vi "一体站氨氮总磷流程平行样自动启动.vi"(11 "参数":T1) -> ()   [LabVIEW 2016, in "质控单元.lvlib"]
panel:
  out "枚举":enum16{"初始化", "采配水启动", "等待", "配水", "排水", "结束"}(ring)
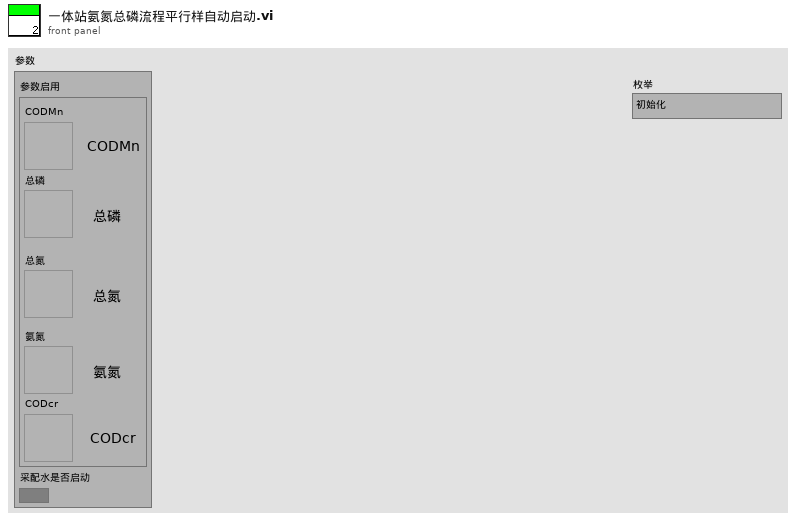
[diagram p1: front panel]
types:
  T1 = cluster{"参数启用":cluster{"CODMn":bool, "总磷":bool, "总氮":bool, "氨氮":bool, "CODcr":bool}, "采配水是否启动":bool}
  T2 = cluster{"命令":string, cluster{"starting address":u16, "holding register value":u16}}
  T3 = typedef "质控单元.lvlib/平行样测试流程.ctl" = enum16{"待机", "第一次水样测试启动", "第一次水样测试中", "第二次水样测试启动", "第二次水样测试中", "存储平行样测试数据", "结束"}
  T4 = cluster{"站号":u16, "量程切换":enum32{"H", "L", "AUTO"}, "控制命令":enum16{"启动测量", "标样核查", "零点核查", "跨度核查", "空白测试", "平行样测试", "加标回收", "空白校准", "标样校准", "初始化（清洗）", "停止测试", "仪器重启", "校时", "模式设置", "测量间隔设置"}, "模式设置":enum16{"待机", "连续模式", "周期模式", "定点模式", "受控模式", "手动模式"}, "测量间隔":u16}
  T5 = cluster{"时间标识":timestamp, "设备":string, "日志信息":string}
  T6 = enum16{"空闲", "水样测试", "标样核查", "零点核查", "跨度核查", "空白测试", "平行样测试", "加标回收", "空白校准", "标样校准", "初始化（清洗）"}
  T7 = cluster{"测量模式":enum16{"水样测量", "标样核查", "零点核查", "跨度核查", "空白测试", "加标回收", "平行样", "校零", "校标"}}
  T8 = cluster{"时间标识":timestamp, "设备":string, "日志信息":string, "流程参数":string}
  T9 = cluster{"R0":i16, "R1":i16, "R2":i16, "R3":i16, "R4":i16, "R5":i16, "R6":i16, "R7":i16, "R8":i16, "R9":i16, "R10":i16, "R11":i16, "R12":i16, "R13":i16, "R14":i16, "R15":i16, "R16":i16, "R17":i16, "R18":i16, "R19":i16, "R20":i16, "R21":i16, "R22":i16, "R23":i16, "R24":i16, "R25":i16, "R26":i16, "R27":i16, "R28":i16, "R29":i16, "R30":i16, "R31":i16, "R32":i16, "R33":i16, "R34":i16, "R35":i16, "R36":i16, "R37":i16, "R38":i16, "R39":i16, "R40":i16, "R41":i16, "R42":i16, "R43":i16, "R44":i16, "R45":i16, "R46":i16, "R47":i16, "R48":i16, "R49":i16, "R50":i16, "R51":i16, "R52":i16, "R53":i16, "R54":i16, "R55":i16, "R56":i16}
  T10 = cluster{"系统时间":timestamp, "工作状态":enum16{"空闲", "水样测试", "标样核查", "零点核查", "跨度核查", "空白测试", "平行样测试", "加标回收", "空白校准", "标样校准", "初始化（清洗）"}, "测量模式":enum16{"待机", "连续模式", "周期模式", "定点模式", "受控模式", "手动模式"}, "告警代码":enum16{"无告警", "缺试剂告警", "缺水样告警", "缺蒸馏水告警", "缺标液告警", "仪表漏液告警", "标定异常告警", "超量程告警", "加热异常", "低试剂预警", "超上限告警", "超下限告警", "仪表内部其他异常", "滴定异常告警", "电极异常告警", "量程切换告警", "参数设置告警", "PH电极电位异常", "电导率电极异常", "浊度光度异常", "溶解氧电极异常", "溶解氧光强异常", "温度异常告警", "PH异常告警", "溶解氧异常告警", "电导率异常告警", "浊度异常告警", "叶绿素异常告警", "藻密度异常告警", "蓝绿藻异常告警", "ORP异常告警", "氨氮异常告警", "清洁刷异常告警", "SD卡异常告警", "蓝牙异常告警", "Wifi异常告警", "流程异常告警"}, "故障代码":enum16{"无故障", "电机故障", "温度故障", "通讯故障", "滴定故障"}, "日志代码":u16, "软件版本":u16, "F0":sgl, "F1":sgl, "F2":sgl, "F3":sgl, "T":sgl, "H":sgl, "id":u16, "flowid":u16, "量程":u16, "总磷控温温度1":sgl, "营养盐控温温度2":sgl, "ADC":sgl}
  T11 = cluster{"因子编码":u32, "单位":u16, "标样参考值":sgl, "水样数据时间":timestamp, "水样实测值":sgl, "水样数据标识":string, "标样数据时间":timestamp, "标样实测值":sgl, "标样数据标识":string, "空白数据时间":timestamp, "空白实测值":sgl, "空白数据标识":string, "零点核查数据时间":timestamp, "零点核查实测值":sgl, "零点核查数据标识":string, "跨度核查数据时间":timestamp, "跨度核查实测值":sgl, "跨度核查数据标识":string, "加标回收数据时间":timestamp, "加标回收实测值":sgl, "加标回收数据标识":string, "平行样数据时间":timestamp, "平行样实测值":sgl, "平行样数据标识":string}
  T12 = cluster{"时间标识":timestamp, "参数":string, "数据类型":string, "第一次水样浓度值":sgl, "第二次水样测试时间":timestamp, "第二次水样浓度值":sgl}
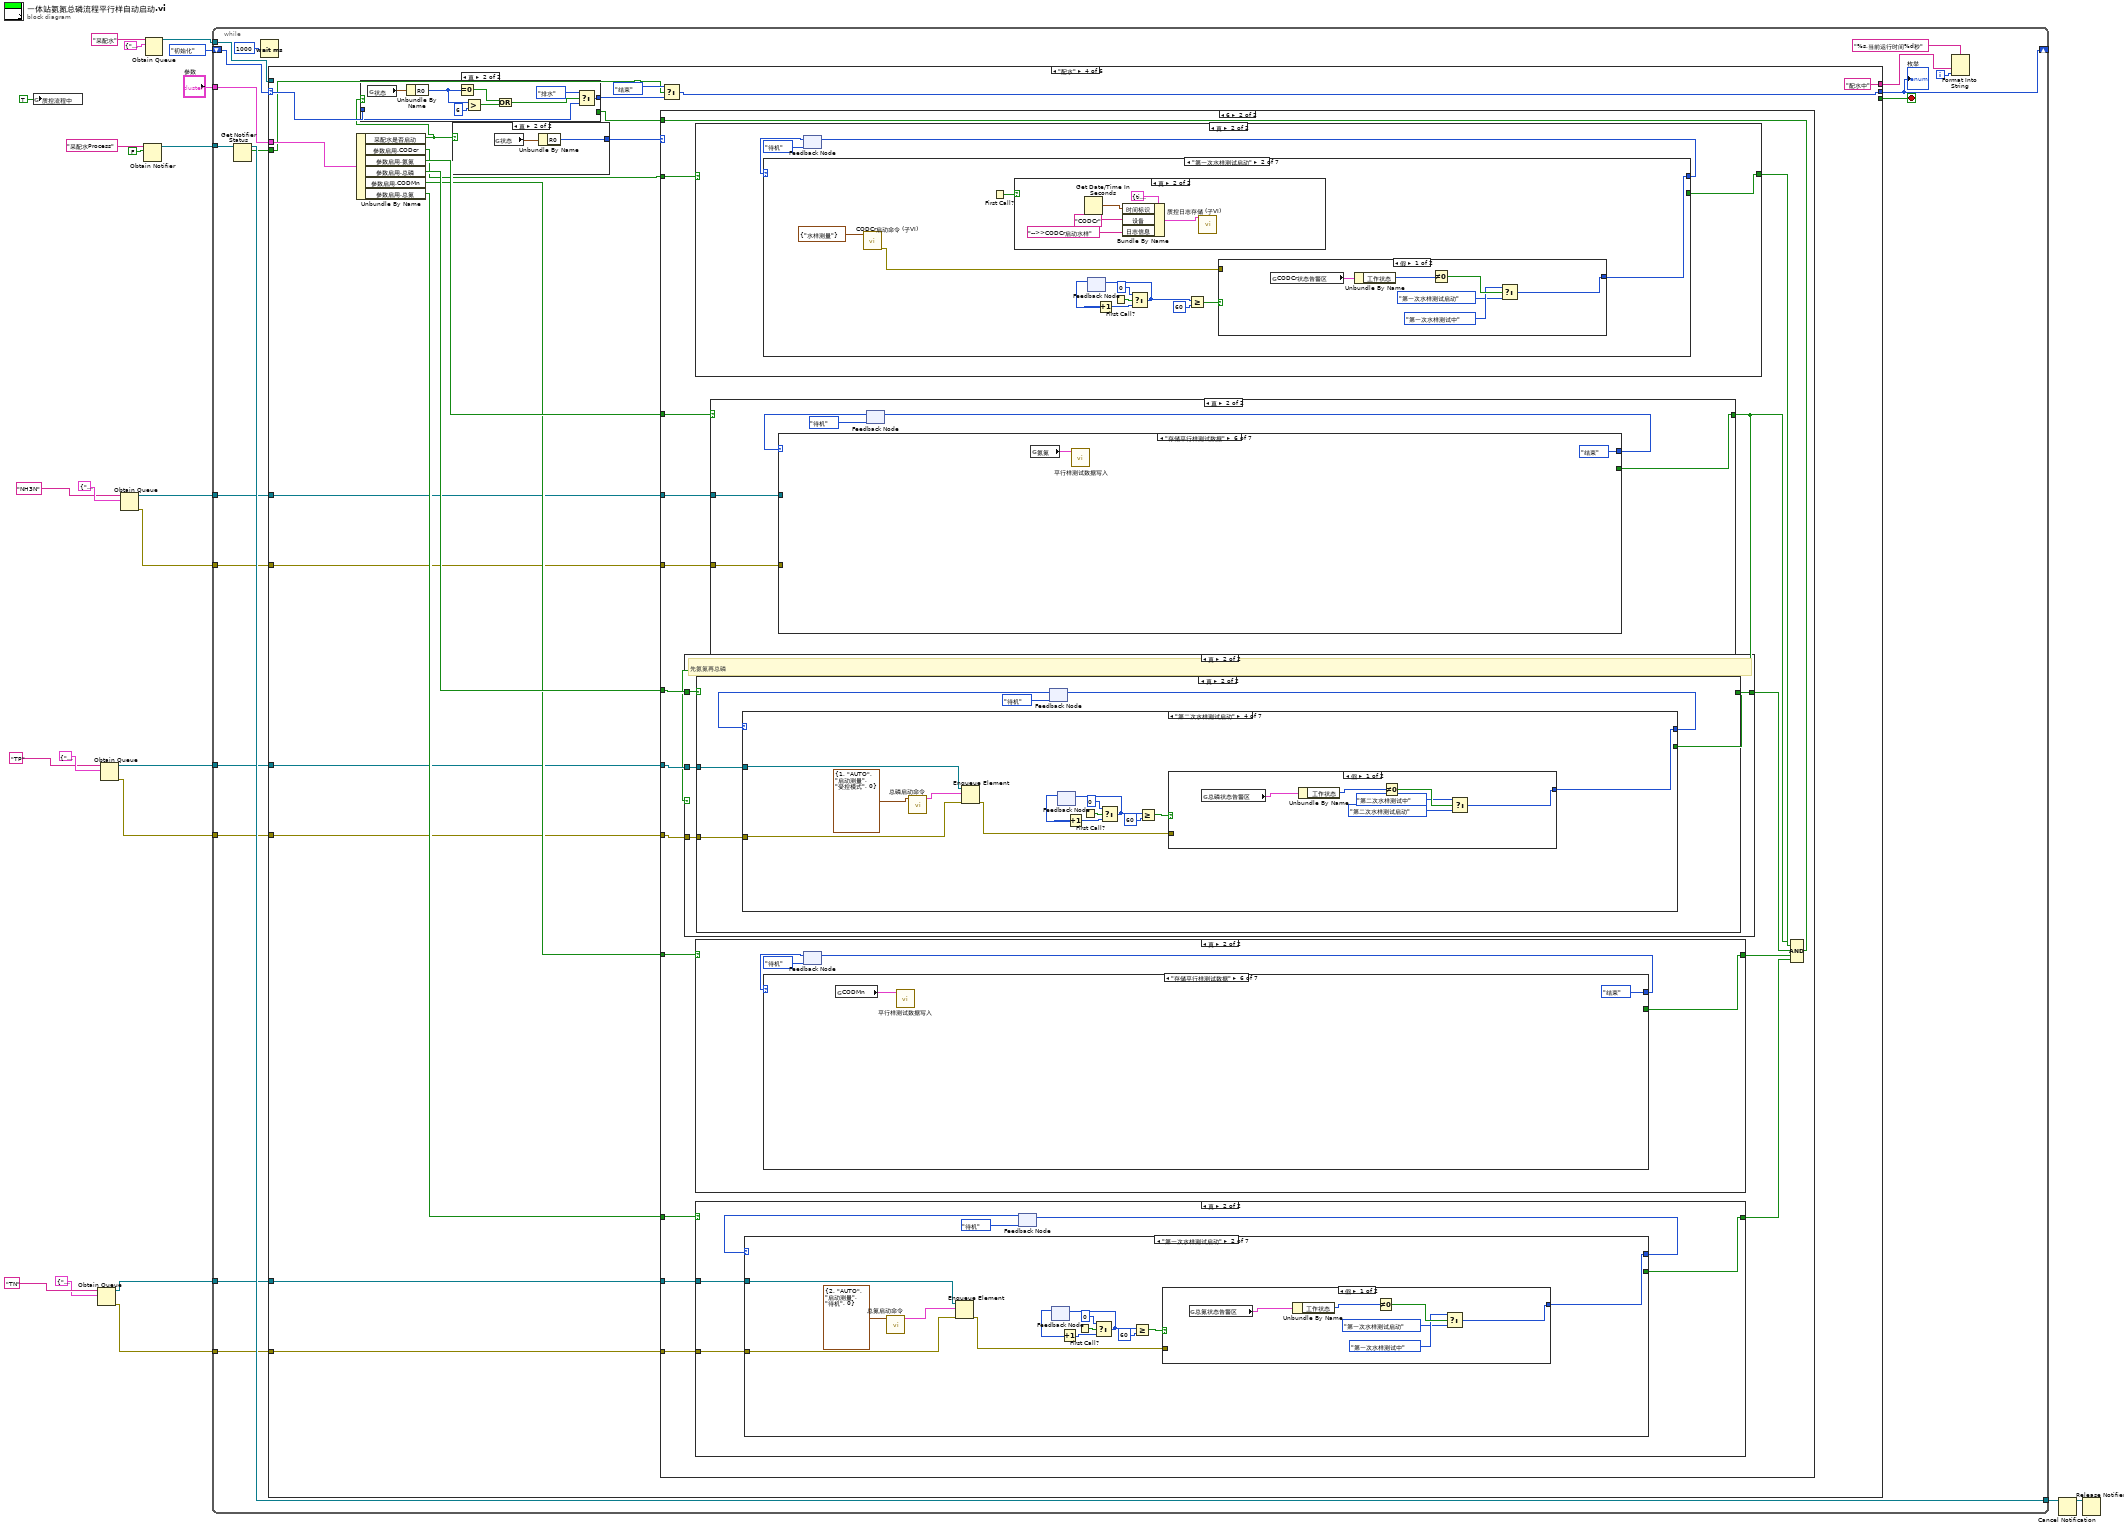
[diagram p0: block diagram]
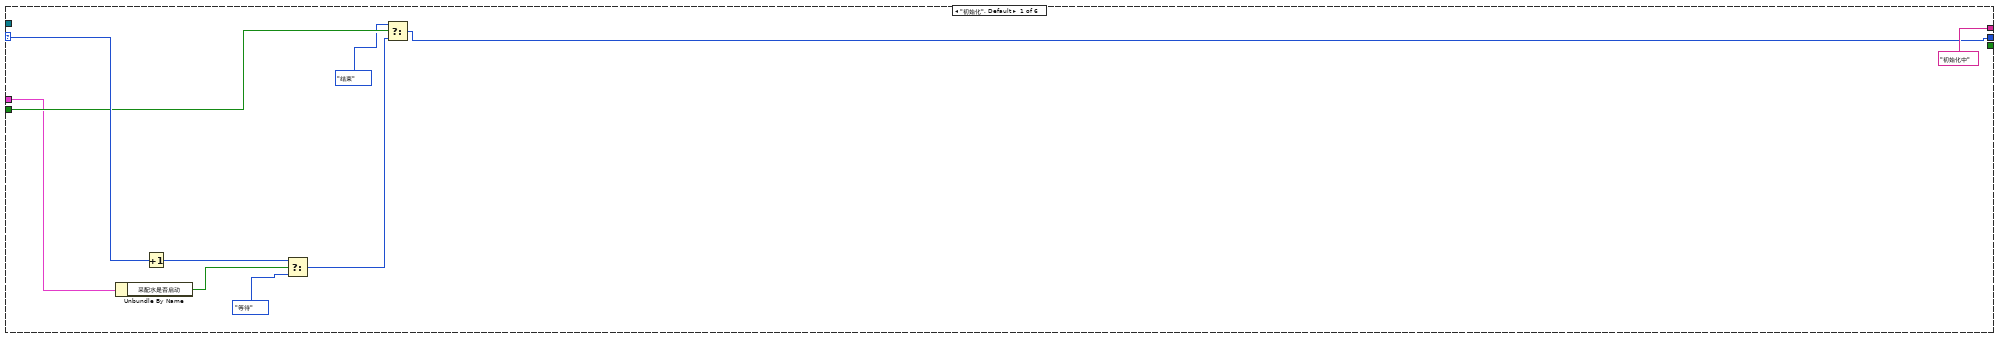
[diagram p2: hidden frame]
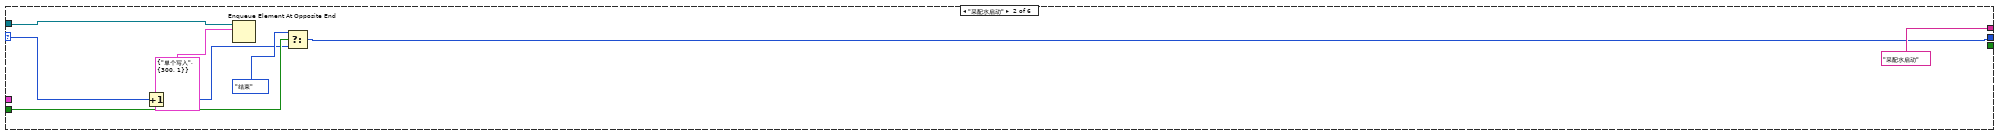
[diagram p3: hidden frame]
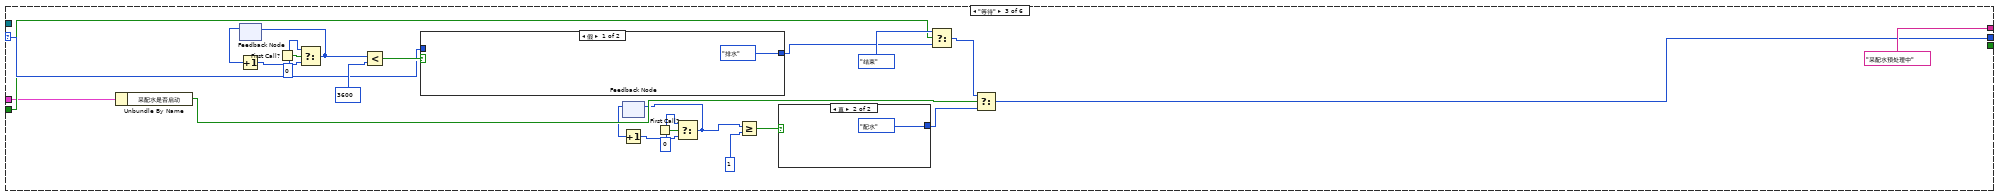
[diagram p4: hidden frame]
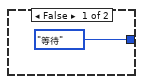
[diagram p5: hidden frame]
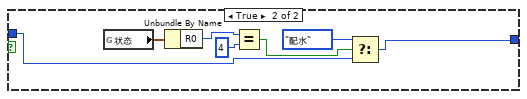
[diagram p6: hidden frame]
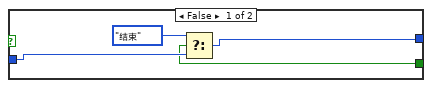
[diagram p7: hidden frame]
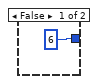
[diagram p8: hidden frame]
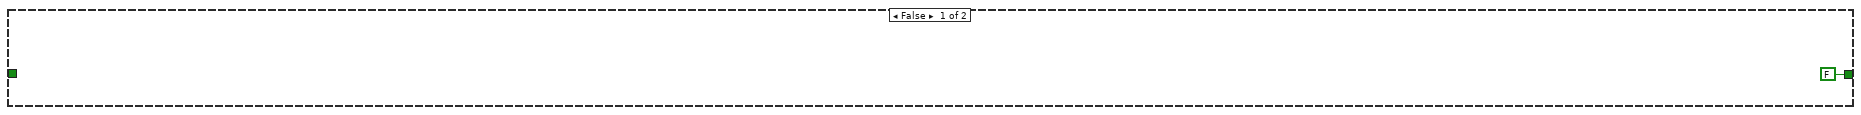
[diagram p10: hidden frame]
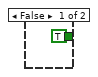
[diagram p11: hidden frame]
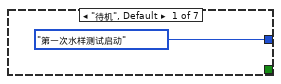
[diagram p12: hidden frame]
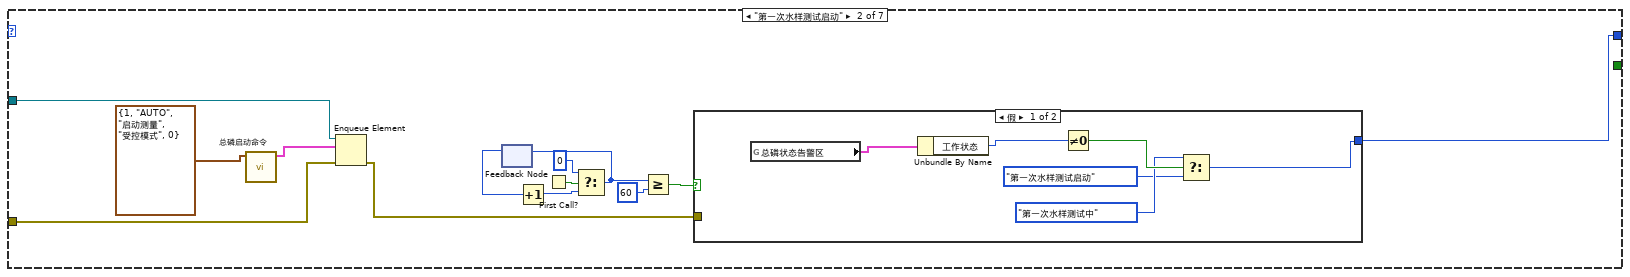
[diagram p13: hidden frame]
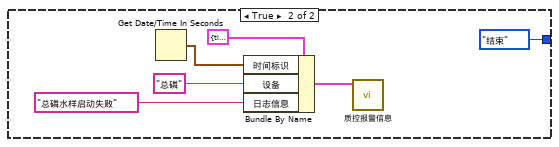
[diagram p14: hidden frame]
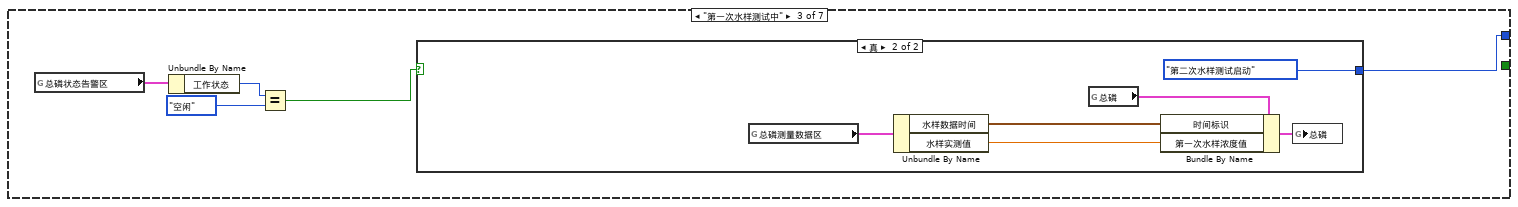
[diagram p15: hidden frame]
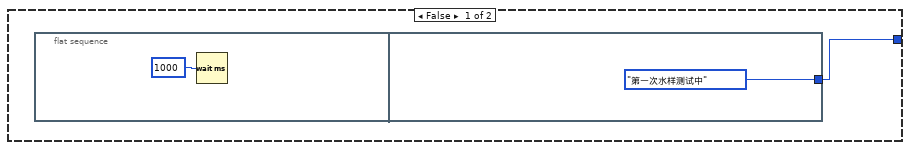
[diagram p16: hidden frame]
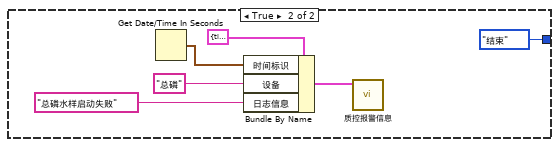
[diagram p17: hidden frame]
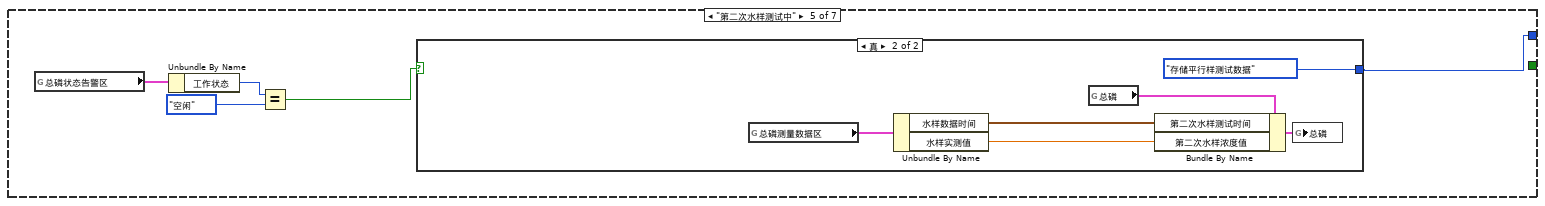
[diagram p18: hidden frame]
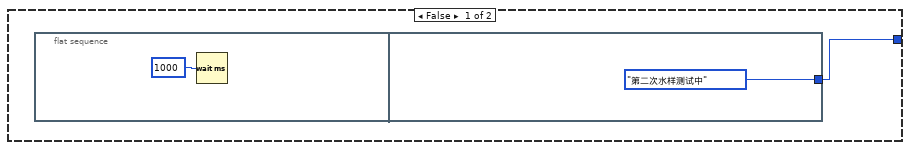
[diagram p19: hidden frame]
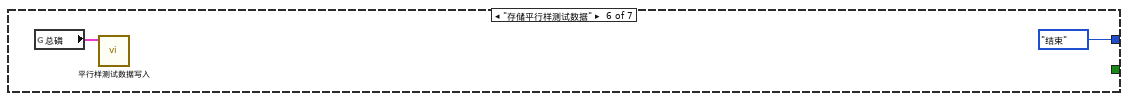
[diagram p20: hidden frame]
diagram:
  n1 = global write "质控测完标志全局 1.vi" "质控流程中"(TRUE ("质控流程中")) -> ()
  n2 = Obtain Queue(name (unnamed)="TN" ("名称（未命名）"), element data type=cluster{"命令":string, "data":variant} {"命令"="", "data"=variant}) -> (queue out=w3:refnum<queue>, error out=w2:errorcluster)  [unwired: 3 in, 1 out]
  n3 = Obtain Queue(name (unnamed)="TP" ("名称（未命名）"), element data type=cluster{"命令":string, "data":variant} {"命令"="", "data"=variant}) -> (queue out=w5:refnum<queue>, error out=w4:errorcluster)  [unwired: 3 in, 1 out]
  n4 = Obtain Queue(name (unnamed)="NH3N" ("名称（未命名）"), element data type=cluster{"命令":string, "data":variant} {"命令"="", "data"=variant}) -> (queue out=w7:refnum<queue>, error out=w6:errorcluster)  [unwired: 3 in, 1 out]
  n5 = Obtain Notifier(name (unnamed)="采配水Process" ("名称（未命名）"), notification data type=FALSE) -> (notifier out=w16:refnum<notifier>)  [unwired: 2 in, 2 out]
  n6 = Obtain Queue(name (unnamed)="采配水" ("名称（未命名）"), element data type=cluster{"命令":string, "数据":variant} {"命令"="", "数据"=variant}) -> (queue out=w21:refnum<queue>)  [unwired: 3 in, 2 out]
  n7 = while {
    tunnel: w21 -> [w41]
    shift-right: [w39] -> _
    shift-left: enum16{"初始化", "采配水启动", "等待", "配水", "排水", "结束"}."初始化" ("枚举") -> [w40]
    tunnel: "参数" -> [w37]
    tunnel: w16 -> [w36]
    tunnel: [w35] -> w15
    tunnel: w7 -> [w30]
    tunnel: w6 -> [w29]
    tunnel: w5 -> [w28]
    tunnel: w4 -> [w27]
    tunnel: w3 -> [w26]
    tunnel: w2 -> [w25]
    i -> [w32]
    stop <- w24 stop-if-true
    n8 = Get Notifier Status(notifier=w36) -> (notifier out=w35:refnum<notifier>, current notification=w31:bool)  [unwired: 1 in, 3 out]
    n9 = Wait (ms)(milliseconds to wait=u32 1000 ("等待时间（毫秒）")) -> ()  [unwired: 1 out]
    n10 = case shown="\"配水\"" w40 {
      selector: w40 -> [w51 w57 w81 w114 w596 w603]
      tunnel: w41 -> [_ w58 _ _ w597 _]
      tunnel: [w48 w52 w60 w111 w591 w602] -> w39
      tunnel: [_ _ _ _ _ TRUE] -> w24
      tunnel: w37 -> [w46 _ w71 w107 _ _]
      tunnel: ["初始化中" ("输入 1") "采配水启动" ("输入 1") "采配水预处理中" ("输入 1") "配水中" ("输入 1") "排水中" ("输入 1") "结束" ("输入 1")] -> w33
      tunnel: w31 -> [w49 w54 w73 w95 w593 _]
      tunnel: w30 -> [_ _ _ w102 _ _]
      tunnel: w29 -> [_ _ _ w101 _ _]
      tunnel: w28 -> [_ _ _ w100 _ _]
      tunnel: w27 -> [_ _ _ w99 _ _]
      tunnel: w26 -> [_ _ _ w98 _ _]
      tunnel: w25 -> [_ _ _ w97 _ _]
      frame "初始化", Default {
        n11 = Unbundle By Name(w46) -> ("采配水是否启动"=w45:bool)
        n12 = Increment(x=w51) -> (x+1=w44:enum16{"初始化", "采配水启动", "等待", "配水", "排水", "结束"})
        n13 = Select(t=w44, s=w45, f=enum16{"初始化", "采配水启动", "等待", "配水", "排水", "结束"}."等待") -> (s? t:f=w43:enum16{"初始化", "采配水启动", "等待", "配水", "排水", "结束"})
        n14 = Select(t=enum16{"初始化", "采配水启动", "等待", "配水", "排水", "结束"}."结束", s=w49, f=w43) -> (s? t:f=w48:enum16{"初始化", "采配水启动", "等待", "配水", "排水", "结束"})
      }
      frame "采配水启动" {
        n15 = Increment(x=w57) -> (x+1=w53:enum16{"初始化", "采配水启动", "等待", "配水", "排水", "结束"})
        n16 = Enqueue Element At Opposite End(queue=w58, element=T2 {"命令"="单个写入", {"starting address"=300, "holding register value"=1}} ("元素")) -> ()  [unwired: 2 in, 3 out]
        n17 = Select(t=enum16{"初始化", "采配水启动", "等待", "配水", "排水", "结束"}."结束", s=w54, f=w53) -> (s? t:f=w52:enum16{"初始化", "采配水启动", "等待", "配水", "排水", "结束"})
      }
      frame "等待" {
        n18 = Unbundle By Name(w71) -> ("采配水是否启动"=w70:bool)
        n19 = feedback #1() -> (w78:i32)  [unwired: 1 in]
        n20 = Increment(x=w78) -> (x+1=w77:i32)
        n21 = First Call?() -> (First Call?: T/F=w79:bool)
        n22 = Select(t=0, s=w79, f=w77) -> (s? t:f=w76:i32)
        n23 = feedback-in #1(w76) -> ()
        n24 = Less?(x=w76, y=3600) -> (x < y?=w82:bool)
        n25 = case shown="假" w82 {
          tunnel: w81 -> [_ w88]
          tunnel: [enum16{"初始化", "采配水启动", "等待", "配水", "排水", "结束"}."排水" ("枚举") w87] -> w72
          frame False {
          }
          frame True {
            n26 = global read "与采配水交互全局.vi" "状态"() -> (w93:T9)
            n27 = Unbundle By Name(w93) -> ("R0"=w92:i16)
            n28 = Equal?(x=w92, y=i16 4) -> (x = y?=w90:bool)
            n29 = Select(t=enum16{"初始化", "采配水启动", "等待", "配水", "排水", "结束"}."配水" ("枚举"), s=w90, f=w88) -> (s? t:f=w87:enum16{"初始化", "采配水启动", "等待", "配水", "排水", "结束"})
          }
        }
        n30 = feedback #2() -> (w66:i32)  [unwired: 1 in]
        n31 = Increment(x=w66) -> (x+1=w67:i32)
        n32 = First Call?() -> (First Call?: T/F=w65:bool)
        n33 = Select(t=0, s=w65, f=w67) -> (s? t:f=w68:i32)
        n34 = feedback-in #2(w68) -> ()
        n35 = Greater Or Equal?(x=w68, y=1) -> (x >= y?=w62:bool)
        n36 = case shown="真" w62 {
          tunnel: [enum16{"初始化", "采配水启动", "等待", "配水", "排水", "结束"}."等待" ("t") enum16{"初始化", "采配水启动", "等待", "配水", "排水", "结束"}."配水" ("t")] -> w61
          frame False {
          }
          frame True {
          }
        }
        n37 = Select(t=enum16{"初始化", "采配水启动", "等待", "配水", "排水", "结束"}."结束", s=w73, f=w72) -> (s? t:f=w69:enum16{"初始化", "采配水启动", "等待", "配水", "排水", "结束"})
        n38 = Select(t=w69, s=w70, f=w61) -> (s? t:f=w60:enum16{"初始化", "采配水启动", "等待", "配水", "排水", "结束"})
      }
      frame "配水" {
        n39 = Unbundle By Name(w107) -> ("采配水是否启动"=w96:bool, "参数启用.CODcr"=w106:bool, "参数启用.氨氮"=w110:bool, "参数启用.总磷"=w109:bool, "参数启用.CODMn"=w108:bool, "参数启用.总氮"=w105:bool)
        n40 = case shown="真" w96 {
          tunnel: [i16 6 ("R0") w129] -> w104
          frame False {
          }
          frame True {
            n41 = global read "与采配水交互全局.vi" "状态"() -> (w130:T9)
            n42 = Unbundle By Name(w130) -> ("R0"=w129:i16)
          }
        }
        n43 = case shown="6" w104 {
          tunnel: w110 -> [_ w147]
          tunnel: w109 -> [_ w146]
          tunnel: w108 -> [_ w145]
          tunnel: w106 -> [_ w144]
          tunnel: w105 -> [_ w141]
          tunnel: w102 -> [_ w139]
          tunnel: w101 -> [_ w138]
          tunnel: w100 -> [_ w137]
          tunnel: w99 -> [_ w136]
          tunnel: w98 -> [_ w135]
          tunnel: w97 -> [_ w134]
          tunnel: [_ w133] -> w94
          frame 0, Default {
          }
          frame 6 {
            n44 = case shown="真" w144 {
              tunnel: [TRUE w498] -> w143
              frame False {
              }
              frame True {
                n45 = feedback #3(平行样测试流程."待机") -> (w500:T3)
                n46 = case shown="\"第一次水样测试启动\"" w500 {
                  tunnel: [平行样测试流程."第一次水样测试启动" w512 w534 w554 w576 平行样测试流程."结束" 平行样测试流程."结束"] -> w499
                  tunnel: [_ _ _ _ _ _ TRUE] -> w498
                  frame "待机", Default {
                  }
                  frame "第一次水样测试启动" {
                    n47 = call "CODCr启动命令 (子VI).vi"("启动测量模式"=T7 {"测量模式"=enum."水样测量"}) -> ("错误输出"=w502:errorcluster)  [unwired: 10 in]
                    n48 = First Call?() -> (First Call?: T/F=w504:bool)
                    n49 = case shown="真" w504 {
                      frame False {
                      }
                      frame True {
                        n50 = Get Date/Time In Seconds() -> (seconds since 1Jan1904=w515:timestamp)
                        n51 = Bundle By Name(cluster=T8 {"时间标识"=timestamp(0 s since 1904-01-01), "设备"="", "日志信息"="", "流程参数"=""} ("data in"), "时间标识"=w515, "设备"="CODCr", "日志信息"="-->>CODCr启动水样") -> (w516:T8)
                        n52 = call "质控日志存储 (子VI).vi"("data in"=w516) -> ()  [unwired: 11 in]
                      }
                    }
                    n53 = feedback #4() -> (w508:i32)  [unwired: 1 in]
                    n54 = Increment(x=w508) -> (x+1=w509:i32)
                    n55 = First Call?() -> (First Call?: T/F=w507:bool)
                    n56 = Select(t=0, s=w507, f=w509) -> (s? t:f=w510:i32)
                    n57 = feedback-in #4(w510) -> ()
                    n58 = Greater Or Equal?(x=w510, y=60) -> (x >= y?=w505:bool)
                    n59 = case shown="假" w505 {
                      tunnel: [w522 平行样测试流程."结束"] -> w512
                      tunnel: w502 -> [_ _]
                      frame False {
                        n60 = global read "与CODCr交互全局.vi" "CODCr状态告警区"() -> (w519:T10)
                        n61 = Unbundle By Name(w519) -> ("工作状态"=w518:T6)
                        n62 = Not Equal To 0?(x=w518) -> (x != 0?=w523:bool)
                        n63 = Select(t=平行样测试流程."第一次水样测试中", s=w523, f=平行样测试流程."第一次水样测试启动") -> (s? t:f=w522:T3)
                      }
                      frame True {
                        n64 = Get Date/Time In Seconds() -> (seconds since 1Jan1904=w526:timestamp)
                        n65 = Bundle By Name(cluster=T5 {"时间标识"=timestamp(0 s since 1904-01-01), "设备"="", "日志信息"=""} ("data in"), "时间标识"=w526, "设备"="CODCr", "日志信息"="CODCr水样启动失败") -> (w524:T5)
                        n66 = call "质控报警信息.vi"("data in"=w524) -> ()  [unwired: 10 in, 1 out]
                      }
                    }
                  }
                  frame "第一次水样测试中" {
                    n67 = global read "与CODCr交互全局.vi" "CODCr状态告警区"() -> (w533:T10)
                    n68 = Unbundle By Name(w533) -> ("工作状态"=w530:T6)
                    n69 = Equal?(x=w530, y=T6."空闲" ("工作状态")) -> (x = y?=w532:bool)
                    n70 = case shown="真" w532 {
                      tunnel: [w535 平行样测试流程."第二次水样测试启动"] -> w534
                      frame False {
                        n71 = flat-sequence {
                          tunnel: [平行样测试流程."第一次水样测试中"] -> w535
                          frame #0 {
                            n72 = Wait (ms)(milliseconds to wait=u32 1000 ("等待时间（毫秒）")) -> ()  [unwired: 1 out]
                          }
                          frame #1 {
                          }
                        }
                      }
                      frame True {
                        n73 = global read "与CODCr交互全局.vi" "CODCr测量数据区"() -> (w540:T11)
                        n74 = Unbundle By Name(w540) -> ("水样数据时间"=w539:timestamp, "水样实测值"=w538:sgl)
                        n75 = global read "平行样测试全局变量.vi" "CODcr"() -> (w542:T12)
                        n76 = Bundle By Name(cluster=w542, "时间标识"=w539, "第一次水样浓度值"=w538) -> (w541:T12)
                        n77 = global write "平行样测试全局变量.vi" "CODcr"(w541) -> ()
                      }
                    }
                  }
                  frame "第二次水样测试启动" {
                    n78 = call "CODCr启动命令 (子VI).vi"("启动测量模式"=T7 {"测量模式"=enum."水样测量"}) -> ("错误输出"=w544:errorcluster)  [unwired: 10 in]
                    n79 = First Call?() -> (First Call?: T/F=w546:bool)
                    n80 = case shown="真" w546 {
                      frame False {
                      }
                      frame True {
                        n81 = Get Date/Time In Seconds() -> (seconds since 1Jan1904=w557:timestamp)
                        n82 = Bundle By Name(cluster=T8 {"时间标识"=timestamp(0 s since 1904-01-01), "设备"="", "日志信息"="", "流程参数"=""} ("data in"), "时间标识"=w557, "设备"="CODCr", "日志信息"="-->>CODCr启动水样") -> (w558:T8)
                        n83 = call "质控日志存储 (子VI).vi"("data in"=w558) -> ()  [unwired: 11 in]
                      }
                    }
                    n84 = First Call?() -> (First Call?: T/F=w549:bool)
                    n85 = feedback #5() -> (w550:i32)  [unwired: 1 in]
                    n86 = Increment(x=w550) -> (x+1=w551:i32)
                    n87 = Select(t=0, s=w549, f=w551) -> (s? t:f=w552:i32)
                    n88 = feedback-in #5(w552) -> ()
                    n89 = Greater Or Equal?(x=w552, y=60) -> (x >= y?=w547:bool)
                    n90 = case shown="假" w547 {
                      tunnel: [w564 平行样测试流程."结束"] -> w554
                      tunnel: w544 -> [_ _]
                      frame False {
                        n91 = global read "与CODCr交互全局.vi" "CODCr状态告警区"() -> (w561:T10)
                        n92 = Unbundle By Name(w561) -> ("工作状态"=w560:T6)
                        n93 = Not Equal To 0?(x=w560) -> (x != 0?=w565:bool)
                        n94 = Select(t=平行样测试流程."第二次水样测试中", s=w565, f=平行样测试流程."第二次水样测试启动") -> (s? t:f=w564:T3)
                      }
                      frame True {
                        n95 = Get Date/Time In Seconds() -> (seconds since 1Jan1904=w568:timestamp)
                        n96 = Bundle By Name(cluster=T5 {"时间标识"=timestamp(0 s since 1904-01-01), "设备"="", "日志信息"=""} ("data in"), "时间标识"=w568, "设备"="CODCr", "日志信息"="CODCr启动失败") -> (w566:T5)
                        n97 = call "质控报警信息.vi"("data in"=w566) -> ()  [unwired: 10 in, 1 out]
                      }
                    }
                  }
                  frame "第二次水样测试中" {
                    n98 = global read "与CODCr交互全局.vi" "CODCr状态告警区"() -> (w575:T10)
                    n99 = Unbundle By Name(w575) -> ("工作状态"=w572:T6)
                    n100 = Equal?(x=w572, y=T6."空闲" ("工作状态")) -> (x = y?=w574:bool)
                    n101 = case shown="假" w574 {
                      tunnel: [w577 平行样测试流程."存储平行样测试数据"] -> w576
                      frame False {
                        n102 = flat-sequence {
                          tunnel: [平行样测试流程."第二次水样测试中"] -> w577
                          frame #0 {
                            n103 = Wait (ms)(milliseconds to wait=u32 1000 ("等待时间（毫秒）")) -> ()  [unwired: 1 out]
                          }
                          frame #1 {
                          }
                        }
                      }
                      frame True {
                        n104 = global read "与CODCr交互全局.vi" "CODCr测量数据区"() -> (w582:T11)
                        n105 = Unbundle By Name(w582) -> ("水样数据时间"=w581:timestamp, "水样实测值"=w580:sgl)
                        n106 = global read "平行样测试全局变量.vi" "CODcr"() -> (w584:T12)
                        n107 = Bundle By Name(cluster=w584, "第二次水样测试时间"=w581, "第二次水样浓度值"=w580) -> (w583:T12)
                        n108 = global write "平行样测试全局变量.vi" "CODcr"(w583) -> ()
                      }
                    }
                  }
                  frame "存储平行样测试数据" {
                    n109 = global read "平行样测试全局变量.vi" "CODcr"() -> (w586:T12)
                    n110 = call "平行样测试数据写入.vi"("data"=w586) -> ()  [unwired: 10 in, 1 out]
                  }
                  frame "结束" {
                    n111 = First Call?() -> (First Call?: T/F=w589:bool)
                    n112 = case shown="真" w589 {
                      frame False {
                      }
                      frame True {
                        (unwired) "-->>CODCr停止" ("日志信息")
                        (unwired) "CODCr" ("设备")
                        n113 = call "质控日志存储 (子VI).vi"() -> ()  [unwired: 12 in]
                      }
                    }
                  }
                }
                n114 = feedback-in #3(w499) -> ()
              }
            }
            n115 = case shown="真" w145 {
              tunnel: [TRUE w424] -> w142
              frame False {
              }
              frame True {
                n116 = feedback #6(平行样测试流程."待机") -> (w426:T3)
                n117 = case shown="\"存储平行样测试数据\"" w426 {
                  tunnel: [平行样测试流程."第一次水样测试启动" w437 w451 w469 w483 平行样测试流程."结束" 平行样测试流程."结束"] -> w425
                  tunnel: [_ _ _ _ _ _ TRUE] -> w424
                  frame "待机", Default {
                  }
                  frame "第一次水样测试启动" {
                    n118 = feedback #7() -> (w433:i32)  [unwired: 1 in]
                    n119 = Increment(x=w433) -> (x+1=w434:i32)
                    n120 = call "CODMn启动命令 (子VI).vi"("启动测量模式"=T7 {"测量模式"=enum."水样测量"}) -> ("错误输出"=w428:errorcluster)  [unwired: 10 in]
                    n121 = First Call?() -> (First Call?: T/F=w432:bool)
                    n122 = Select(t=0, s=w432, f=w434) -> (s? t:f=w435:i32)
                    n123 = feedback-in #7(w435) -> ()
                    n124 = Greater Or Equal?(x=w435, y=60) -> (x >= y?=w430:bool)
                    n125 = case shown="真" w430 {
                      tunnel: [w441 平行样测试流程."结束"] -> w437
                      tunnel: w428 -> [_ _]
                      frame False {
                        n126 = global read "与CODMn交互全局.vi" "多列列表框"() -> (w440:i32)
                        n127 = Not Equal To 0?(x=w440) -> (x != 0?=w442:bool)
                        n128 = Select(t=平行样测试流程."第一次水样测试中", s=w442, f=平行样测试流程."第一次水样测试启动") -> (s? t:f=w441:T3)
                      }
                      frame True {
                        n129 = Get Date/Time In Seconds() -> (seconds since 1Jan1904=w445:timestamp)
                        n130 = Bundle By Name(cluster=T5 {"时间标识"=timestamp(0 s since 1904-01-01), "设备"="", "日志信息"=""} ("data in"), "时间标识"=w445, "设备"="CODMn", "日志信息"="CODMn启动失败") -> (w443:T5)
                        n131 = call "质控报警信息.vi"("data in"=w443) -> ()  [unwired: 10 in, 1 out]
                      }
                    }
                  }
                  frame "第一次水样测试中" {
                    n132 = global read "与CODMn交互全局.vi" "多列列表框"() -> (w450:i32)
                    n133 = Equal To 0?(x=w450) -> (x = 0?=w449:bool)
                    n134 = case shown="假" w449 {
                      tunnel: [w452 平行样测试流程."第二次水样测试启动"] -> w451
                      frame False {
                        n135 = flat-sequence {
                          tunnel: [平行样测试流程."第一次水样测试中"] -> w452
                          frame #0 {
                            n136 = Wait (ms)(milliseconds to wait=u32 1000 ("等待时间（毫秒）")) -> ()  [unwired: 1 out]
                          }
                          frame #1 {
                          }
                        }
                      }
                      frame True {
                        n137 = global read "与CODMn交互全局.vi" "COD浓度（mg/L)"() -> (w455:dbl)
                        n138 = global read "与CODMn交互全局.vi" "水样启动时间"() -> (w456:timestamp)
                        n139 = global read "平行样测试全局变量.vi" "CODMn"() -> (w458:T12)
                        n140 = Bundle By Name(cluster=w458, "时间标识"=w456, "第一次水样浓度值"=w455) -> (w457:T12)
                        n141 = global write "平行样测试全局变量.vi" "CODMn"(w457) -> ()
                      }
                    }
                  }
                  frame "第二次水样测试启动" {
                    n142 = feedback #8() -> (w465:i32)  [unwired: 1 in]
                    n143 = Increment(x=w465) -> (x+1=w466:i32)
                    n144 = First Call?() -> (First Call?: T/F=w464:bool)
                    n145 = call "CODMn启动命令 (子VI).vi"("启动测量模式"=T7 {"测量模式"=enum."水样测量"}) -> ("错误输出"=w460:errorcluster)  [unwired: 10 in]
                    n146 = Select(t=0, s=w464, f=w466) -> (s? t:f=w467:i32)
                    n147 = feedback-in #8(w467) -> ()
                    n148 = Greater Or Equal?(x=w467, y=60) -> (x >= y?=w462:bool)
                    n149 = case shown="真" w462 {
                      tunnel: [w473 平行样测试流程."结束"] -> w469
                      tunnel: w460 -> [_ _]
                      frame False {
                        n150 = global read "与CODMn交互全局.vi" "多列列表框"() -> (w472:i32)
                        n151 = Not Equal To 0?(x=w472) -> (x != 0?=w474:bool)
                        n152 = Select(t=平行样测试流程."第二次水样测试中", s=w474, f=平行样测试流程."第二次水样测试启动") -> (s? t:f=w473:T3)
                      }
                      frame True {
                        n153 = Get Date/Time In Seconds() -> (seconds since 1Jan1904=w477:timestamp)
                        n154 = Bundle By Name(cluster=T5 {"时间标识"=timestamp(0 s since 1904-01-01), "设备"="", "日志信息"=""} ("data in"), "时间标识"=w477, "设备"="CODMn", "日志信息"="CODMn启动失败") -> (w475:T5)
                        n155 = call "质控报警信息.vi"("data in"=w475) -> ()  [unwired: 10 in, 1 out]
                      }
                    }
                  }
                  frame "第二次水样测试中" {
                    n156 = global read "与CODMn交互全局.vi" "多列列表框"() -> (w482:i32)
                    n157 = Equal To 0?(x=w482) -> (x = 0?=w481:bool)
                    n158 = case shown="真" w481 {
                      tunnel: [w484 平行样测试流程."存储平行样测试数据"] -> w483
                      frame False {
                        n159 = flat-sequence {
                          tunnel: [平行样测试流程."第二次水样测试中"] -> w484
                          frame #0 {
                            n160 = Wait (ms)(milliseconds to wait=u32 1000 ("等待时间（毫秒）")) -> ()  [unwired: 1 out]
                          }
                          frame #1 {
                          }
                        }
                      }
                      frame True {
                        n161 = global read "与CODMn交互全局.vi" "COD浓度（mg/L)"() -> (w487:dbl)
                        n162 = global read "与CODMn交互全局.vi" "水样启动时间"() -> (w488:timestamp)
                        n163 = global read "平行样测试全局变量.vi" "CODMn"() -> (w490:T12)
                        n164 = Bundle By Name(cluster=w490, "时间标识"=w488, "第一次水样浓度值"=w487) -> (w489:T12)
                        n165 = global write "平行样测试全局变量.vi" "CODMn"(w489) -> ()
                      }
                    }
                  }
                  frame "存储平行样测试数据" {
                    n166 = global read "平行样测试全局变量.vi" "CODMn"() -> (w492:T12)
                    n167 = call "平行样测试数据写入.vi"("data"=w492) -> ()  [unwired: 10 in, 1 out]
                  }
                  frame "结束" {
                  }
                }
                n168 = feedback-in #6(w425) -> ()
              }
            }
            n169 = case shown="真" w141 {
              tunnel: [TRUE w336] -> w140
              tunnel: w135 -> [_ w334]
              tunnel: w134 -> [_ w333]
              frame False {
              }
              frame True {
                n170 = feedback #9(平行样测试流程."待机") -> (w338:T3)
                n171 = case shown="\"第一次水样测试启动\"" w338 {
                  tunnel: [平行样测试流程."第一次水样测试启动" w340 w366 w379 w404 平行样测试流程."结束" 平行样测试流程."结束"] -> w337
                  tunnel: [_ _ _ _ _ _ TRUE] -> w336
                  tunnel: w334 -> [_ w344 _ w381 _ _ _]
                  tunnel: w333 -> [_ w343 _ w380 _ _ _]
                  frame "待机", Default {
                  }
                  frame "第一次水样测试启动" {
                    n172 = call "总氮启动命令.vi"("参数"=T4 {"站号"=2, "量程切换"=enum."AUTO", "控制命令"=enum."启动测量", "模式设置"=enum."待机", "测量间隔"=0}) -> ("启动命令"=w342:cluster{"命令":string, "data":variant})  [unwired: 10 in]
                    n173 = Enqueue Element(queue=w344, element=w342, error in (no error)=w343) -> (error out=w345:errorcluster)  [unwired: 1 in, 2 out]
                    n174 = feedback #10() -> (w349:i32)  [unwired: 1 in]
                    n175 = Increment(x=w349) -> (x+1=w348:i32)
                    n176 = First Call?() -> (First Call?: T/F=w350:bool)
                    n177 = Select(t=0, s=w350, f=w348) -> (s? t:f=w347:i32)
                    n178 = feedback-in #10(w347) -> ()
                    n179 = Greater Or Equal?(x=w347, y=60) -> (x >= y?=w352:bool)
                    n180 = case shown="假" w352 {
                      tunnel: [w357 平行样测试流程."结束"] -> w340
                      tunnel: w345 -> [_ _]
                      frame False {
                        n181 = global read "与总氮交互全局.vi" "总氮状态告警区"() -> (w353:T10)
                        n182 = Unbundle By Name(w353) -> ("工作状态"=w354:T6)
                        n183 = Not Equal To 0?(x=w354) -> (x != 0?=w358:bool)
                        n184 = Select(t=平行样测试流程."第一次水样测试中", s=w358, f=平行样测试流程."第一次水样测试启动") -> (s? t:f=w357:T3)
                      }
                      frame True {
                        n185 = Get Date/Time In Seconds() -> (seconds since 1Jan1904=w361:timestamp)
                        n186 = Bundle By Name(cluster=T5 {"时间标识"=timestamp(0 s since 1904-01-01), "设备"="", "日志信息"=""} ("data in"), "时间标识"=w361, "设备"="总氮", "日志信息"="总氮水样启动失败") -> (w359:T5)
                        n187 = call "质控报警信息.vi"("data in"=w359) -> ()  [unwired: 10 in, 1 out]
                      }
                    }
                  }
                  frame "第一次水样测试中" {
                    n188 = global read "与总氮交互全局.vi" "总氮状态告警区"() -> (w365:T10)
                    n189 = Unbundle By Name(w365) -> ("工作状态"=w369:T6)
                    n190 = Equal?(x=w369, y=T6."空闲" ("工作状态")) -> (x = y?=w367:bool)
                    n191 = case shown="真" w367 {
                      tunnel: [w370 平行样测试流程."第二次水样测试启动"] -> w366
                      frame False {
                        n192 = flat-sequence {
                          tunnel: [平行样测试流程."第一次水样测试中"] -> w370
                          frame #0 {
                            n193 = Wait (ms)(milliseconds to wait=u32 1000 ("等待时间（毫秒）")) -> ()  [unwired: 1 out]
                          }
                          frame #1 {
                          }
                        }
                      }
                      frame True {
                        n194 = global read "与总氮交互全局.vi" "总氮测量数据区"() -> (w373:T11)
                        n195 = Unbundle By Name(w373) -> ("水样数据时间"=w376:timestamp, "水样实测值"=w377:sgl)
                        n196 = global read "平行样测试全局变量.vi" "总氮"() -> (w374:T12)
                        n197 = Bundle By Name(cluster=w374, "时间标识"=w376, "第一次水样浓度值"=w377) -> (w375:T12)
                        n198 = global write "平行样测试全局变量.vi" "总氮"(w375) -> ()
                      }
                    }
                  }
                  frame "第二次水样测试启动" {
                    n199 = call "总氮启动命令.vi"("参数"=T4 {"站号"=2, "量程切换"=enum."AUTO", "控制命令"=enum."启动测量", "模式设置"=enum."待机", "测量间隔"=0}) -> ("启动命令"=w383:cluster{"命令":string, "data":variant})  [unwired: 10 in]
                    n200 = Enqueue Element(queue=w381, element=w383, error in (no error)=w380) -> (error out=w384:errorcluster)  [unwired: 1 in, 2 out]
                    n201 = feedback #11() -> (w388:i32)  [unwired: 1 in]
                    n202 = Increment(x=w388) -> (x+1=w387:i32)
                    n203 = First Call?() -> (First Call?: T/F=w389:bool)
                    n204 = Select(t=0, s=w389, f=w387) -> (s? t:f=w386:i32)
                    n205 = feedback-in #11(w386) -> ()
                    n206 = Greater Or Equal?(x=w386, y=60) -> (x >= y?=w391:bool)
                    n207 = case shown="假" w391 {
                      tunnel: [w396 平行样测试流程."结束"] -> w379
                      tunnel: w384 -> [_ _]
                      frame False {
                        n208 = global read "与总氮交互全局.vi" "总氮状态告警区"() -> (w392:T10)
                        n209 = Unbundle By Name(w392) -> ("工作状态"=w393:T6)
                        n210 = Not Equal To 0?(x=w393) -> (x != 0?=w397:bool)
                        n211 = Select(t=平行样测试流程."第二次水样测试中", s=w397, f=平行样测试流程."第二次水样测试启动") -> (s? t:f=w396:T3)
                      }
                      frame True {
                        n212 = Get Date/Time In Seconds() -> (seconds since 1Jan1904=w400:timestamp)
                        n213 = Bundle By Name(cluster=T5 {"时间标识"=timestamp(0 s since 1904-01-01), "设备"="", "日志信息"=""} ("data in"), "时间标识"=w400, "设备"="总氮", "日志信息"="总氮水样启动失败") -> (w398:T5)
                        n214 = call "质控报警信息.vi"("data in"=w398) -> ()  [unwired: 10 in, 1 out]
                      }
                    }
                  }
                  frame "第二次水样测试中" {
                    n215 = global read "与总氮交互全局.vi" "总氮状态告警区"() -> (w405:T10)
                    n216 = Unbundle By Name(w405) -> ("工作状态"=w408:T6)
                    n217 = Equal?(x=w408, y=T6."空闲" ("工作状态")) -> (x = y?=w406:bool)
                    n218 = case shown="真" w406 {
                      tunnel: [w409 平行样测试流程."存储平行样测试数据"] -> w404
                      frame False {
                        n219 = flat-sequence {
                          tunnel: [平行样测试流程."第二次水样测试中"] -> w409
                          frame #0 {
                            n220 = Wait (ms)(milliseconds to wait=u32 1000 ("等待时间（毫秒）")) -> ()  [unwired: 1 out]
                          }
                          frame #1 {
                          }
                        }
                      }
                      frame True {
                        n221 = global read "与总氮交互全局.vi" "总氮测量数据区"() -> (w412:T11)
                        n222 = Unbundle By Name(w412) -> ("水样数据时间"=w415:timestamp, "水样实测值"=w416:sgl)
                        n223 = global read "平行样测试全局变量.vi" "总氮"() -> (w413:T12)
                        n224 = Bundle By Name(cluster=w413, "第二次水样测试时间"=w415, "第二次水样浓度值"=w416) -> (w414:T12)
                        n225 = global write "平行样测试全局变量.vi" "总氮"(w414) -> ()
                      }
                    }
                  }
                  frame "存储平行样测试数据" {
                    n226 = global read "平行样测试全局变量.vi" "总氮"() -> (w418:T12)
                    n227 = call "平行样测试数据写入.vi"("data"=w418) -> ()  [unwired: 10 in, 1 out]
                  }
                  frame "结束" {
                  }
                }
                n228 = feedback-in #9(w337) -> ()
              }
            }
            n229 = case shown="真" w147 {
              tunnel: [TRUE w246] -> w131
              tunnel: w139 -> [_ w245]
              tunnel: w138 -> [_ w244]
              frame False {
              }
              frame True {
                n230 = feedback #12(平行样测试流程."待机") -> (w248:T3)
                n231 = case shown="\"存储平行样测试数据\"" w248 {
                  tunnel: [平行样测试流程."第一次水样测试启动" w251 w280 w294 w318 平行样测试流程."结束" 平行样测试流程."结束"] -> w247
                  tunnel: [_ _ _ _ _ _ TRUE] -> w246
                  tunnel: w245 -> [_ w261 _ w291 _ _ _]
                  tunnel: w244 -> [_ w260 _ w290 _ _ _]
                  frame "待机", Default {
                  }
                  frame "第一次水样测试启动" {
                    n232 = call "氨氮启动命令.vi"("参数"=T4 {"站号"=3, "量程切换"=enum."AUTO", "控制命令"=enum."启动测量", "模式设置"=enum."受控模式", "测量间隔"=0}) -> ("启动命令"=w263:cluster{"命令":string, "data":variant})  [unwired: 10 in]
                    n233 = Enqueue Element(queue=w261, element=w263, error in (no error)=w260) -> (error out=w252:errorcluster)  [unwired: 1 in, 2 out]
                    n234 = feedback #13() -> (w256:i32)  [unwired: 1 in]
                    n235 = Increment(x=w256) -> (x+1=w257:i32)
                    n236 = First Call?() -> (First Call?: T/F=w255:bool)
                    n237 = Select(t=0, s=w255, f=w257) -> (s? t:f=w258:i32)
                    n238 = feedback-in #13(w258) -> ()
                    n239 = Greater Or Equal?(x=w258, y=60) -> (x >= y?=w253:bool)
                    n240 = case shown="假" w253 {
                      tunnel: [w268 平行样测试流程."结束"] -> w251
                      tunnel: w252 -> [_ _]
                      frame False {
                        n241 = global read "与氨氮交互全局.vi" "氨氮状态告警区"() -> (w264:T10)
                        n242 = Unbundle By Name(w264) -> ("工作状态"=w265:T6)
                        n243 = Not Equal To 0?(x=w265) -> (x != 0?=w269:bool)
                        n244 = Select(t=平行样测试流程."第一次水样测试中", s=w269, f=平行样测试流程."第一次水样测试启动") -> (s? t:f=w268:T3)
                      }
                      frame True {
                        n245 = Get Date/Time In Seconds() -> (seconds since 1Jan1904=w272:timestamp)
                        n246 = Bundle By Name(cluster=T5 {"时间标识"=timestamp(0 s since 1904-01-01), "设备"="", "日志信息"=""} ("data in"), "时间标识"=w272, "设备"="氨氮", "日志信息"="氨氮水样启动失败") -> (w270:T5)
                        n247 = call "质控报警信息.vi"("data in"=w270) -> ()  [unwired: 10 in, 1 out]
                      }
                    }
                  }
                  frame "第一次水样测试中" {
                    n248 = global read "与氨氮交互全局.vi" "氨氮状态告警区"() -> (w279:T10)
                    n249 = Unbundle By Name(w279) -> ("工作状态"=w277:T6)
                    n250 = Equal?(x=w277, y=T6."空闲" ("工作状态")) -> (x = y?=w276:bool)
                    n251 = case shown="真" w276 {
                      tunnel: [w281 平行样测试流程."第二次水样测试启动"] -> w280
                      frame False {
                        n252 = flat-sequence {
                          tunnel: [平行样测试流程."第一次水样测试中"] -> w281
                          frame #0 {
                            n253 = Wait (ms)(milliseconds to wait=u32 1000 ("等待时间（毫秒）")) -> ()  [unwired: 1 out]
                          }
                          frame #1 {
                          }
                        }
                      }
                      frame True {
                        n254 = global read "与氨氮交互全局.vi" "氨氮测量数据区"() -> (w286:T11)
                        n255 = Unbundle By Name(w286) -> ("水样数据时间"=w285:timestamp, "水样实测值"=w284:sgl)
                        n256 = global read "平行样测试全局变量.vi" "氨氮"() -> (w288:T12)
                        n257 = Bundle By Name(cluster=w288, "时间标识"=w285, "第一次水样浓度值"=w284) -> (w287:T12)
                        n258 = global write "平行样测试全局变量.vi" "氨氮"(w287) -> ()
                      }
                    }
                  }
                  frame "第二次水样测试启动" {
                    n259 = call "氨氮启动命令.vi"("参数"=T4 {"站号"=3, "量程切换"=enum."AUTO", "控制命令"=enum."启动测量", "模式设置"=enum."受控模式", "测量间隔"=0}) -> ("启动命令"=w293:cluster{"命令":string, "data":variant})  [unwired: 10 in]
                    n260 = Enqueue Element(queue=w291, element=w293, error in (no error)=w290) -> ()  [unwired: 1 in, 3 out]
                    n261 = feedback #14() -> (w298:i32)  [unwired: 1 in]
                    n262 = Increment(x=w298) -> (x+1=w299:i32)
                    n263 = First Call?() -> (First Call?: T/F=w297:bool)
                    n264 = Select(t=0, s=w297, f=w299) -> (s? t:f=w300:i32)
                    n265 = feedback-in #14(w300) -> ()
                    n266 = Greater Or Equal?(x=w300, y=60) -> (x >= y?=w295:bool)
                    n267 = case shown="假" w295 {
                      tunnel: [w304 平行样测试流程."结束"] -> w294
                      frame False {
                        n268 = global read "与氨氮交互全局.vi" "氨氮状态告警区"() -> (w307:T10)
                        n269 = Unbundle By Name(w307) -> ("工作状态"=w303:T6)
                        n270 = Not Equal To 0?(x=w303) -> (x != 0?=w302:bool)
                        n271 = Select(t=平行样测试流程."第二次水样测试中", s=w302, f=平行样测试流程."第二次水样测试启动") -> (s? t:f=w304:T3)
                      }
                      frame True {
                        n272 = Get Date/Time In Seconds() -> (seconds since 1Jan1904=w310:timestamp)
                        n273 = Bundle By Name(cluster=T5 {"时间标识"=timestamp(0 s since 1904-01-01), "设备"="", "日志信息"=""} ("data in"), "时间标识"=w310, "设备"="氨氮", "日志信息"="氨氮水样启动失败") -> (w309:T5)
                        n274 = call "质控报警信息.vi"("data in"=w309) -> ()  [unwired: 10 in, 1 out]
                      }
                    }
                  }
                  frame "第二次水样测试中" {
                    n275 = global read "与氨氮交互全局.vi" "氨氮状态告警区"() -> (w317:T10)
                    n276 = Unbundle By Name(w317) -> ("工作状态"=w315:T6)
                    n277 = Equal?(x=w315, y=T6."空闲" ("工作状态")) -> (x = y?=w314:bool)
                    n278 = case shown="真" w314 {
                      tunnel: [w319 平行样测试流程."存储平行样测试数据"] -> w318
                      frame False {
                        n279 = flat-sequence {
                          tunnel: [平行样测试流程."第二次水样测试中"] -> w319
                          frame #0 {
                            n280 = Wait (ms)(milliseconds to wait=u32 1000 ("等待时间（毫秒）")) -> ()  [unwired: 1 out]
                          }
                          frame #1 {
                          }
                        }
                      }
                      frame True {
                        n281 = global read "与氨氮交互全局.vi" "氨氮测量数据区"() -> (w324:T11)
                        n282 = Unbundle By Name(w324) -> ("水样数据时间"=w323:timestamp, "水样实测值"=w322:sgl)
                        n283 = global read "平行样测试全局变量.vi" "氨氮"() -> (w326:T12)
                        n284 = Bundle By Name(cluster=w326, "第二次水样测试时间"=w323, "第二次水样浓度值"=w322) -> (w325:T12)
                        n285 = global write "平行样测试全局变量.vi" "氨氮"(w325) -> ()
                      }
                    }
                  }
                  frame "存储平行样测试数据" {
                    n286 = global read "平行样测试全局变量.vi" "氨氮"() -> (w328:T12)
                    n287 = call "平行样测试数据写入.vi"("data"=w328) -> ()  [unwired: 10 in, 1 out]
                  }
                  frame "结束" {
                  }
                }
                n288 = feedback-in #12(w247) -> ()
              }
            }
            n289 = case shown="真" w131 {
              tunnel: w146 -> [_ w152]
              tunnel: w137 -> [_ w151]
              tunnel: w136 -> [_ w150]
              tunnel: [FALSE w149] -> w132
              frame False {
              }
              frame True {
                # "先氨氮再总磷"
                n290 = case shown="真" w152 {
                  tunnel: [TRUE w157] -> w149
                  tunnel: w151 -> [_ w155]
                  tunnel: w150 -> [_ w154]
                  frame False {
                  }
                  frame True {
                    n291 = feedback #15(平行样测试流程."待机") -> (w159:T3)
                    n292 = case shown="\"第二次水样测试启动\"" w159 {
                      tunnel: [平行样测试流程."第一次水样测试启动" w161 w190 w200 w225 平行样测试流程."结束" 平行样测试流程."结束"] -> w158
                      tunnel: [_ _ _ _ _ _ TRUE] -> w157
                      tunnel: w155 -> [_ w173 _ w202 _ _ _]
                      tunnel: w154 -> [_ w172 _ w201 _ _ _]
                      frame "待机", Default {
                      }
                      frame "第一次水样测试启动" {
                        n293 = call "总磷启动命令.vi"("参数"=T4 {"站号"=1, "量程切换"=enum."AUTO", "控制命令"=enum."启动测量", "模式设置"=enum."受控模式", "测量间隔"=0}) -> ("启动命令"=w171:cluster{"命令":string, "data":variant})  [unwired: 10 in]
                        n294 = Enqueue Element(queue=w173, element=w171, error in (no error)=w172) -> (error out=w162:errorcluster)  [unwired: 1 in, 2 out]
                        n295 = feedback #16() -> (w166:i32)  [unwired: 1 in]
                        n296 = Increment(x=w166) -> (x+1=w165:i32)
                        n297 = First Call?() -> (First Call?: T/F=w167:bool)
                        n298 = Select(t=0, s=w167, f=w165) -> (s? t:f=w164:i32)
                        n299 = feedback-in #16(w164) -> ()
                        n300 = Greater Or Equal?(x=w164, y=60) -> (x >= y?=w169:bool)
                        n301 = case shown="假" w169 {
                          tunnel: [w178 平行样测试流程."结束"] -> w161
                          tunnel: w162 -> [_ _]
                          frame False {
                            n302 = global read "与总磷交互全局.vi" "总磷状态告警区"() -> (w174:T10)
                            n303 = Unbundle By Name(w174) -> ("工作状态"=w175:T6)
                            n304 = Not Equal To 0?(x=w175) -> (x != 0?=w179:bool)
                            n305 = Select(t=平行样测试流程."第一次水样测试中", s=w179, f=平行样测试流程."第一次水样测试启动") -> (s? t:f=w178:T3)
                          }
                          frame True {
                            n306 = Get Date/Time In Seconds() -> (seconds since 1Jan1904=w182:timestamp)
                            n307 = Bundle By Name(cluster=T5 {"时间标识"=timestamp(0 s since 1904-01-01), "设备"="", "日志信息"=""} ("data in"), "时间标识"=w182, "设备"="总磷", "日志信息"="总磷水样启动失败") -> (w180:T5)
                            n308 = call "质控报警信息.vi"("data in"=w180) -> ()  [unwired: 10 in, 1 out]
                          }
                        }
                      }
                      frame "第一次水样测试中" {
                        n309 = global read "与总磷交互全局.vi" "总磷状态告警区"() -> (w186:T10)
                        n310 = Unbundle By Name(w186) -> ("工作状态"=w189:T6)
                        n311 = Equal?(x=w189, y=T6."空闲" ("工作状态")) -> (x = y?=w187:bool)
                        n312 = case shown="真" w187 {
                          tunnel: [w191 平行样测试流程."第二次水样测试启动"] -> w190
                          frame False {
                            n313 = flat-sequence {
                              tunnel: [平行样测试流程."第一次水样测试中"] -> w191
                              frame #0 {
                                n314 = Wait (ms)(milliseconds to wait=u32 1000 ("等待时间（毫秒）")) -> ()  [unwired: 1 out]
                              }
                              frame #1 {
                              }
                            }
                          }
                          frame True {
                            n315 = global read "与总磷交互全局.vi" "总磷测量数据区"() -> (w194:T11)
                            n316 = Unbundle By Name(w194) -> ("水样数据时间"=w197:timestamp, "水样实测值"=w198:sgl)
                            n317 = global read "平行样测试全局变量.vi" "总磷"() -> (w195:T12)
                            n318 = Bundle By Name(cluster=w195, "时间标识"=w197, "第一次水样浓度值"=w198) -> (w196:T12)
                            n319 = global write "平行样测试全局变量.vi" "总磷"(w196) -> ()
                          }
                        }
                      }
                      frame "第二次水样测试启动" {
                        n320 = call "总磷启动命令.vi"("参数"=T4 {"站号"=1, "量程切换"=enum."AUTO", "控制命令"=enum."启动测量", "模式设置"=enum."受控模式", "测量间隔"=0}) -> ("启动命令"=w212:cluster{"命令":string, "data":variant})  [unwired: 10 in]
                        n321 = Enqueue Element(queue=w202, element=w212, error in (no error)=w201) -> (error out=w203:errorcluster)  [unwired: 1 in, 2 out]
                        n322 = feedback #17() -> (w207:i32)  [unwired: 1 in]
                        n323 = Increment(x=w207) -> (x+1=w206:i32)
                        n324 = First Call?() -> (First Call?: T/F=w208:bool)
                        n325 = Select(t=0, s=w208, f=w206) -> (s? t:f=w205:i32)
                        n326 = feedback-in #17(w205) -> ()
                        n327 = Greater Or Equal?(x=w205, y=60) -> (x >= y?=w210:bool)
                        n328 = case shown="假" w210 {
                          tunnel: [w217 平行样测试流程."结束"] -> w200
                          tunnel: w203 -> [_ _]
                          frame False {
                            n329 = global read "与总磷交互全局.vi" "总磷状态告警区"() -> (w213:T10)
                            n330 = Unbundle By Name(w213) -> ("工作状态"=w214:T6)
                            n331 = Not Equal To 0?(x=w214) -> (x != 0?=w218:bool)
                            n332 = Select(t=平行样测试流程."第二次水样测试中", s=w218, f=平行样测试流程."第二次水样测试启动") -> (s? t:f=w217:T3)
                          }
                          frame True {
                            n333 = Get Date/Time In Seconds() -> (seconds since 1Jan1904=w221:timestamp)
                            n334 = Bundle By Name(cluster=T5 {"时间标识"=timestamp(0 s since 1904-01-01), "设备"="", "日志信息"=""} ("data in"), "时间标识"=w221, "设备"="总磷", "日志信息"="总磷水样启动失败") -> (w219:T5)
                            n335 = call "质控报警信息.vi"("data in"=w219) -> ()  [unwired: 10 in, 1 out]
                          }
                        }
                      }
                      frame "第二次水样测试中" {
                        n336 = global read "与总磷交互全局.vi" "总磷状态告警区"() -> (w226:T10)
                        n337 = Unbundle By Name(w226) -> ("工作状态"=w229:T6)
                        n338 = Equal?(x=w229, y=T6."空闲" ("工作状态")) -> (x = y?=w227:bool)
                        n339 = case shown="真" w227 {
                          tunnel: [w230 平行样测试流程."存储平行样测试数据"] -> w225
                          frame False {
                            n340 = flat-sequence {
                              tunnel: [平行样测试流程."第二次水样测试中"] -> w230
                              frame #0 {
                                n341 = Wait (ms)(milliseconds to wait=u32 1000 ("等待时间（毫秒）")) -> ()  [unwired: 1 out]
                              }
                              frame #1 {
                              }
                            }
                          }
                          frame True {
                            n342 = global read "与总磷交互全局.vi" "总磷测量数据区"() -> (w233:T11)
                            n343 = Unbundle By Name(w233) -> ("水样数据时间"=w236:timestamp, "水样实测值"=w237:sgl)
                            n344 = global read "平行样测试全局变量.vi" "总磷"() -> (w234:T12)
                            n345 = Bundle By Name(cluster=w234, "第二次水样测试时间"=w236, "第二次水样浓度值"=w237) -> (w235:T12)
                            n346 = global write "平行样测试全局变量.vi" "总磷"(w235) -> ()
                          }
                        }
                      }
                      frame "存储平行样测试数据" {
                        n347 = global read "平行样测试全局变量.vi" "总磷"() -> (w239:T12)
                        n348 = call "平行样测试数据写入.vi"("data"=w239) -> ()  [unwired: 10 in, 1 out]
                      }
                      frame "结束" {
                      }
                    }
                    n349 = feedback-in #15(w158) -> ()
                  }
                }
              }
            }
            n350 = Compound Arithmetic op=AND ("复合运算")(w131, w143, w132, w142, w140) -> (w133:bool)
          }
        }
        n351 = case shown="真" w96 {
          tunnel: w114 -> [w117 w126]
          tunnel: [w116 w125] -> w112
          tunnel: w94 -> [w115 _]
          frame False {
            n352 = Select(t=enum16{"初始化", "采配水启动", "等待", "配水", "排水", "结束"}."结束" ("枚举"), s=w115, f=w117) -> (s? t:f=w116:enum16{"初始化", "采配水启动", "等待", "配水", "排水", "结束"})
          }
          frame True {
            n353 = global read "与采配水交互全局.vi" "状态"() -> (w124:T9)
            n354 = Unbundle By Name(w124) -> ("R0"=w123:i16)
            n355 = Equal To 0?(x=w123) -> (x = 0?=w120:bool)
            n356 = Greater?(x=w123, y=i16 6) -> (0:w121:bool)
            n357 = Or(x=w120, y=w121) -> (x .or. y?=w119:bool)
            n358 = Select(t=enum16{"初始化", "采配水启动", "等待", "配水", "排水", "结束"}."排水" ("枚举"), s=w119, f=w126) -> (s? t:f=w125:enum16{"初始化", "采配水启动", "等待", "配水", "排水", "结束"})
          }
        }
        n359 = Select(t=enum16{"初始化", "采配水启动", "等待", "配水", "排水", "结束"}."结束", s=w95, f=w112) -> (s? t:f=w111:enum16{"初始化", "采配水启动", "等待", "配水", "排水", "结束"})
      }
      frame "排水" {
        n360 = Increment(x=w596) -> (x+1=w592:enum16{"初始化", "采配水启动", "等待", "配水", "排水", "结束"})
        n361 = Enqueue Element At Opposite End(queue=w597, element=T2 {"命令"="单个写入", {"starting address"=303, "holding register value"=1}} ("元素")) -> ()  [unwired: 2 in, 3 out]
        n362 = Select(t=enum16{"初始化", "采配水启动", "等待", "配水", "排水", "结束"}."结束", s=w593, f=w592) -> (s? t:f=w591:enum16{"初始化", "采配水启动", "等待", "配水", "排水", "结束"})
      }
      frame "结束" {
        n363 = Increment(x=w603) -> (x+1=w602:enum16{"初始化", "采配水启动", "等待", "配水", "排水", "结束"})
        n364 = global write "质控测完标志全局 1.vi" "质控流程中"(FALSE ("质控流程中")) -> ()
      }
    }
    "枚举" <- w39
    n365 = Format Into String(format string="%s,当前运行时间%d秒" ("格式字符串"), w33, w32) -> ()  [unwired: 2 in, 2 out]
  }
  n366 = Cancel Notification(0:w15) -> (8:w14:refnum<notifier>)  [unwired: 1 in, 2 out]
  n367 = Release Notifier(notifier=w14) -> ()  [unwired: 2 in, 3 out]
